vi "get_image_resolution.vi"(8 "error in (no error)":errorcluster, 11 "ScanModeMG091111IntrinsicImaging in":refnum<class "ImagingModeMG091111IntrinsicImaging.lvclass">) -> (0 "error out":errorcluster, 1 "ImageHeight":i32, 2 "ImageWidth":i32, 3 "ScanModeMG091111IntrinsicImaging out":refnum<class "ImagingModeMG091111IntrinsicImaging.lvclass">)   [LabVIEW 2010, in "ImagingModeMG091111IntrinsicImaging.lvclass"]
uses:
  ImagingModeMG091111IntrinsicImaging.lvclass
  ImagingModeMG091111IntrinsicImaging.lvclass/ImagingModeMG091111IntrinsicImaging.ctl
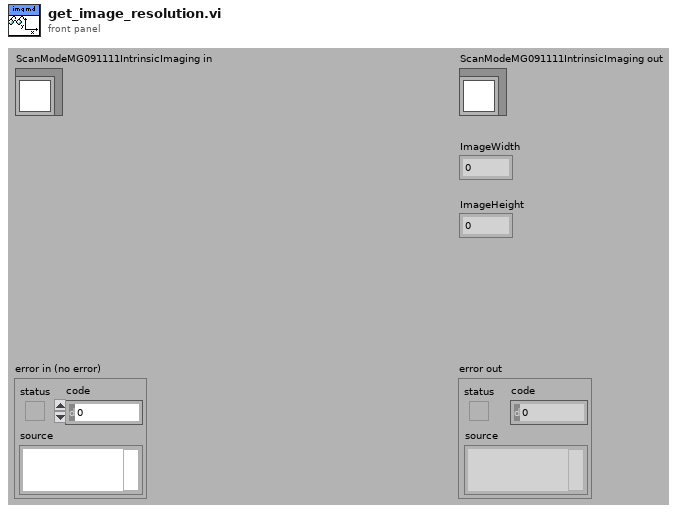
[diagram p1: front panel]
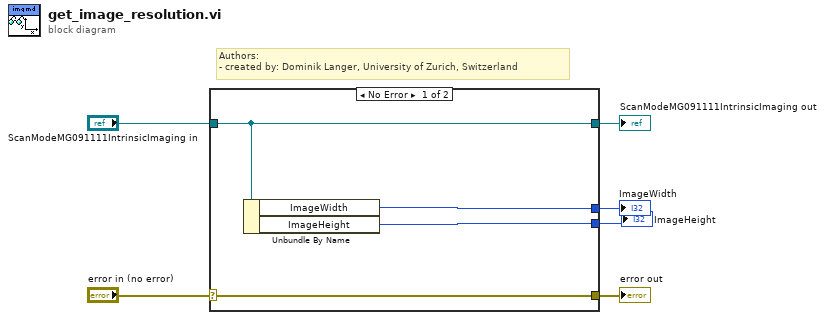
[diagram p0: block diagram]
diagram:
  # "Authors: \n- created by: Dominik Langer, University of Zurich, Switzerland"
  n1 = case shown="No Error" "error in (no error)" {
    selector: "error in (no error)" -> [w10 w11]
    tunnel: [w10 w11] -> w5
    tunnel: [w9 w12] -> w3
    tunnel: "ScanModeMG091111IntrinsicImaging in" -> [w9 w12]
    tunnel: [w8 _] -> w2
    tunnel: [w7 _] -> w1
    frame No Error {
      n2 = Unbundle By Name(w9) -> ("ImageWidth"=w8:i32, "ImageHeight"=w7:i32)
    }
    frame Error {
    }
  }
  "error out" <- w5
  "ScanModeMG091111IntrinsicImaging out" <- w3
  "ImageWidth" <- w2
  "ImageHeight" <- w1
